vi "Write Deviated Values.vi"(8 "Error in":errorcluster, 10 "Deviated Values":dbl[](array[numeric]), 11 "Device in":refnum<class "Device.lvclass">) -> (0 "Error out":errorcluster, 3 "Device out":refnum<class "Device.lvclass">)   [LabVIEW 2020, in "Device.lvclass"]
uses:
  Device.lvclass
  Device.lvclass/Device.ctl
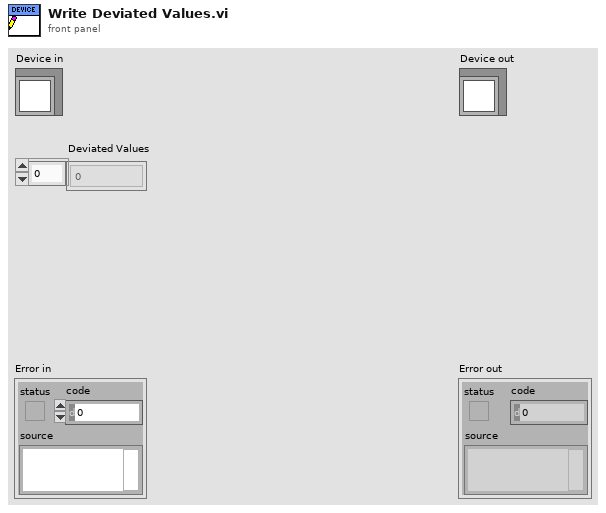
[diagram p1: front panel]
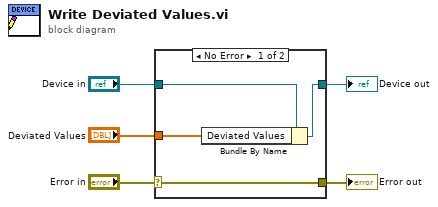
[diagram p0: block diagram]
diagram:
  n1 = case shown="No Error" "Error in" {
    selector: "Error in" -> [w9 w10]
    tunnel: [w9 w10] -> w4
    tunnel: [w7 w11] -> w2
    tunnel: "Device in" -> [w8 w11]
    tunnel: "Deviated Values" -> [w6 _]
    frame No Error {
      n2 = Bundle By Name(cluster=w8, "Deviated Values"=w6) -> (w7:refnum<class "Device.lvclass">)
    }
    frame Error {
    }
  }
  "Error out" <- w4
  "Device out" <- w2
